vi "Level-Enumerate Valid Params.vi"(8 "error in (no error)":errorcluster, 11 "Level":T2(xcontrol)) -> (0 "error out":errorcluster, 2 "Parameter Names":string[](array[string]))   [LabVIEW 2015]
uses:
  Level XCtl.xctl
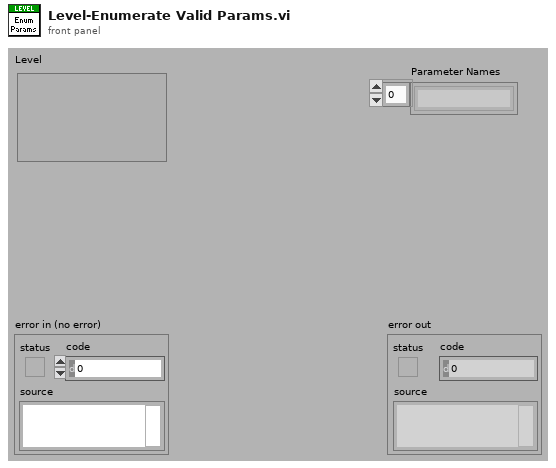
[diagram p1: front panel]
types:
  T1 = typedef "Level Units.ctl" = enum16{"dB atten", "dB SPL", "dB re 1 Vrms", "dB V/Hz½", "mW", "dB SL"}
  T2 = cluster{"Level":dbl, "Units":T1, "Max":dbl, "Multiplier":dbl, "Cal File":path, "Cal":cluster{"Freq (Hz)":dbl[], "Mag (dB SPL)":dbl[], "Phase (deg)":dbl[]}}
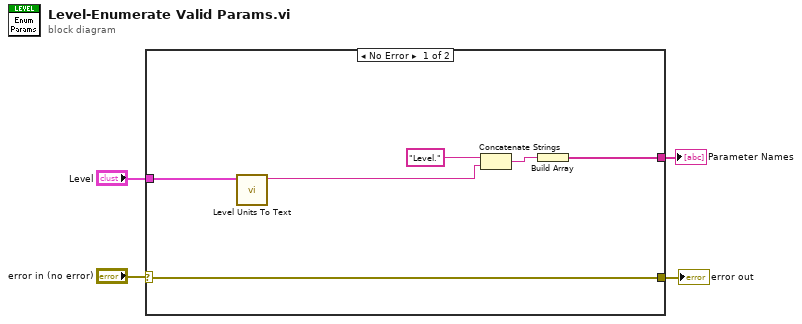
[diagram p0: block diagram]
diagram:
  n1 = case shown="No Error" "error in (no error)" {
    selector: "error in (no error)" -> [w10 w11]
    tunnel: "Level" -> [w7 _]
    tunnel: [w10 w11] -> w2
    tunnel: [w8 _] -> w1
    frame No Error {
      n2 = call "Level Units To Text.vi"("Level"=w7) -> ("String"=w5:string)  [unwired: 9 in, 1 out]
      n3 = Concatenate Strings("Level.", w5) -> (w6:string)
      n4 = Build Array(w6) -> (w8:string[])
    }
    frame Error {
    }
  }
  "error out" <- w2
  "Parameter Names" <- w1
